vi "Vision On.vi"() -> ()   [LabVIEW 2019]
panel:
  in  "Vision On":bool
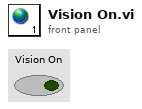
[diagram p1: front panel]
diagram:
